vi "标样核查数据发送(子VI).vi"   [LabVIEW 2016, in "数据传输系统-02.lvlib"]
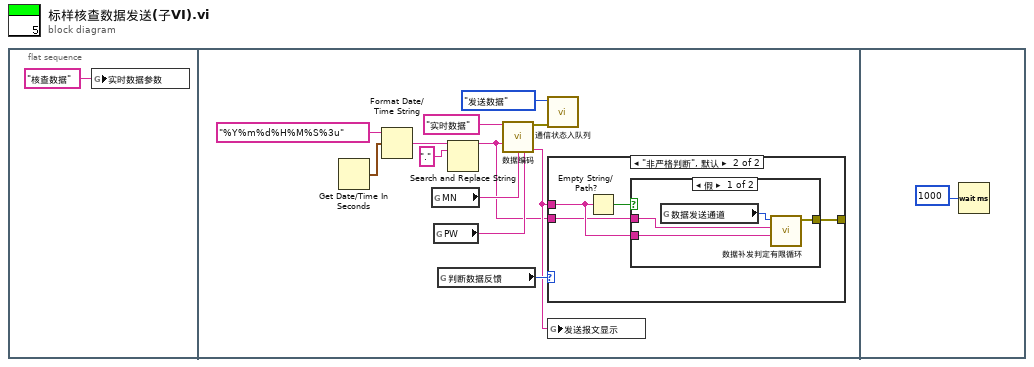
[diagram p0: block diagram]
diagram:
  n1 = flat-sequence {
    frame #0 {
      n2 = global write "全局 实时数据参数.vi" "实时数据参数"("核查数据") -> ()
    }
    frame #1 {
      n3 = Get Date/Time In Seconds() -> (seconds since 1Jan1904=w11:timestamp)
      n4 = Format Date/Time String(time format string (%c)="%Y%m%d%H%M%S%3u" ("时间格式字符串(%c)"), seconds (now)=w11) -> (date/time string=w12:string)  [unwired: 1 in]
      n5 = global read "断电保存全局.vi" "MN"() -> (w7:string)
      n6 = global read "断电保存全局.vi" "PW"() -> (w8:string)
      n7 = global read "断电保存全局.vi" "判断数据反馈"() -> (w4:enum16{"非严格判断", "严格判断", "不判断"})
      n8 = Search and Replace String(input string=w12, search string="." ("搜索字符串")) -> (result string=w2:string)  [unwired: 6 in, 3 out]
      n9 = call "数据编码.vi"("table输入"="实时数据" ("新元素/子数组"), "QN"=w2, "MN"=w7, "PW"=w8) -> ("错误常量"=w9:errorcluster, "通讯包字符串"=w3:string)  [unwired: 10 in]
      n10 = call "通信状态入队列.vi"("错误输入（无错误）"=w9, "枚举"=enum16{"打开连接", "发送数据", "读取数据", "数据处理", "关闭连接"}."发送数据") -> ()  [unwired: 9 in, 1 out]
      n11 = case shown="\"非严格判断\", 默认" w4 {
        tunnel: [_ w17] -> _
        tunnel: w3 -> [_ w16]
        tunnel: w2 -> [_ w15]
        frame "不判断" {
        }
        frame "非严格判断", Default {
          n12 = Empty String/Path?(string/path=w16) -> (empty?=w14:bool)
          n13 = case shown="假" w14 {
            tunnel: [w21 _] -> w17
            tunnel: w16 -> [w20 _]
            tunnel: w15 -> [w18 _]
            frame False {
              n14 = global read "断电保存全局.vi" "数据发送通道"() -> (w19:enum16{"TCP", "VISA"})
              n15 = call "数据补发判定有限循环.vi"("数据输入"=w20, "QN"=w18, "数据发送通道"=w19) -> ("error out"=w21:errorcluster)  [unwired: 8 in]
            }
            frame True {
            }
          }
        }
      }
      n16 = global write "全局1.vi" "发送报文显示"(w3) -> ()
    }
    frame #2 {
      n17 = Wait (ms)(milliseconds to wait=u32 1000 ("等待时间（毫秒）")) -> ()  [unwired: 1 out]
    }
  }
